vi "Ohaus (com6).vi"(4 "State":i16, 5 "Time":dbl format="%.2f", 6 "Sensor Values":dbl[](array[numeric]), 7 "Set Points":dbl[](array[numeric])) -> (0 "required data":T1, 3 "output value":dbl)   [LabVIEW 2015]
uses:
  <vilib>/Instr/_visa.llb/VISA Configure Serial Port (Instr).vi
panel:
  out "VISA resource name out":refnum<visa-resource-name>
  # "Enter the correct information for this control code in the required data structure below. Then make the current value default by right clicking on the border of the data structure. Select \"data operations\" and then select \"make current value default\". These values will be displayed by process controller."
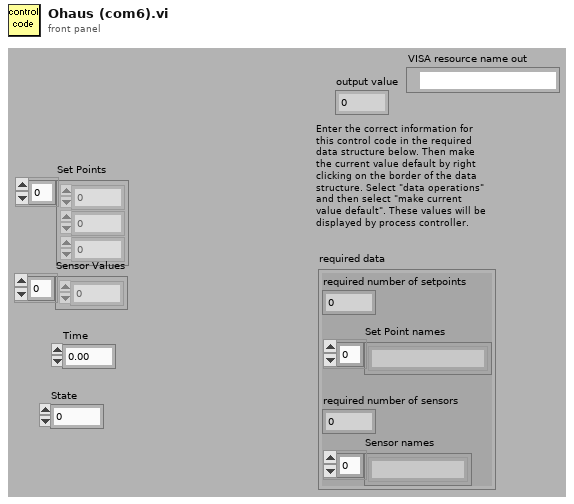
[diagram p1: front panel]
types:
  T1 = cluster{"Set Point names":string[], "required number of setpoints":u8, "required number of sensors":u8, "Sensor names":string[]}
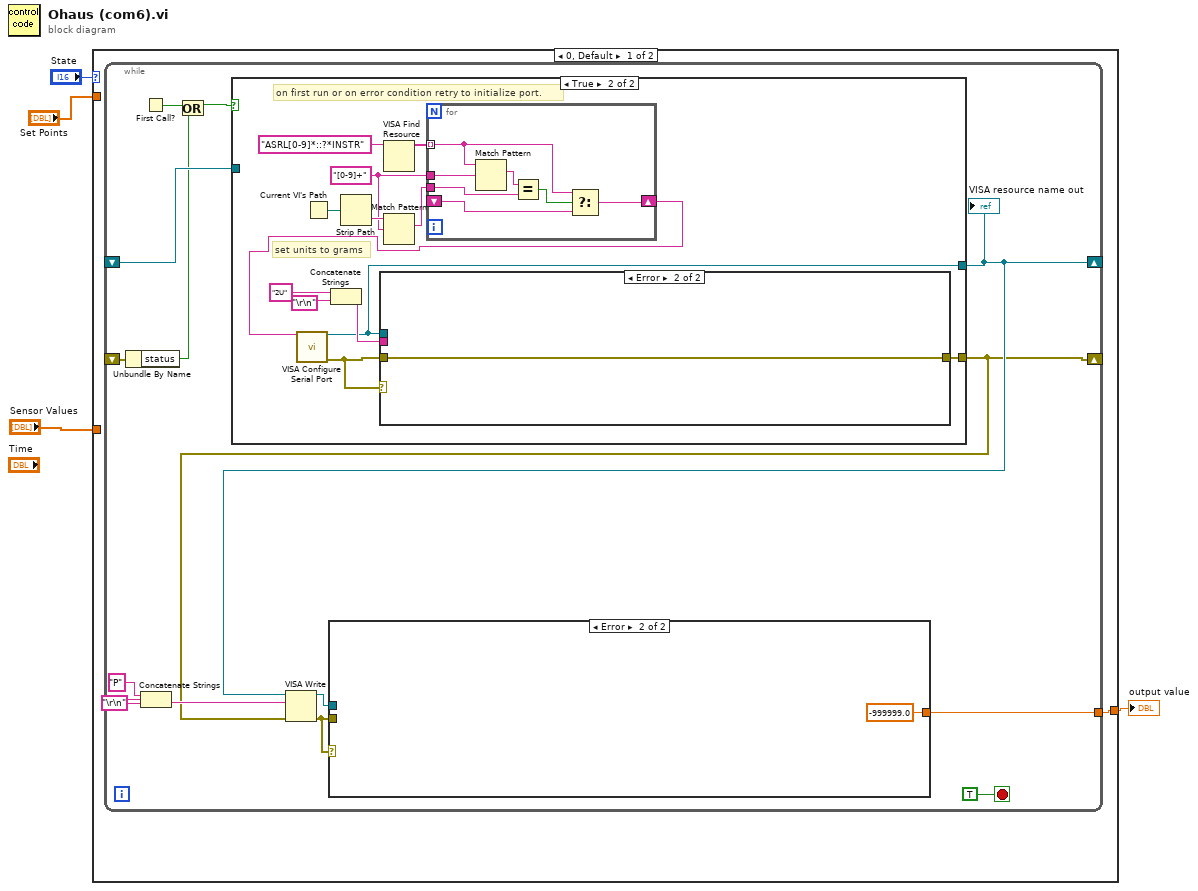
[diagram p0: block diagram]
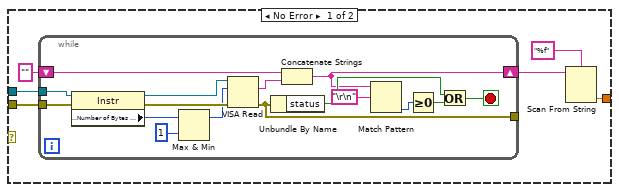
[diagram p2: hidden frame]
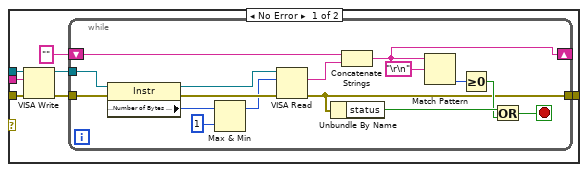
[diagram p4: hidden frame]
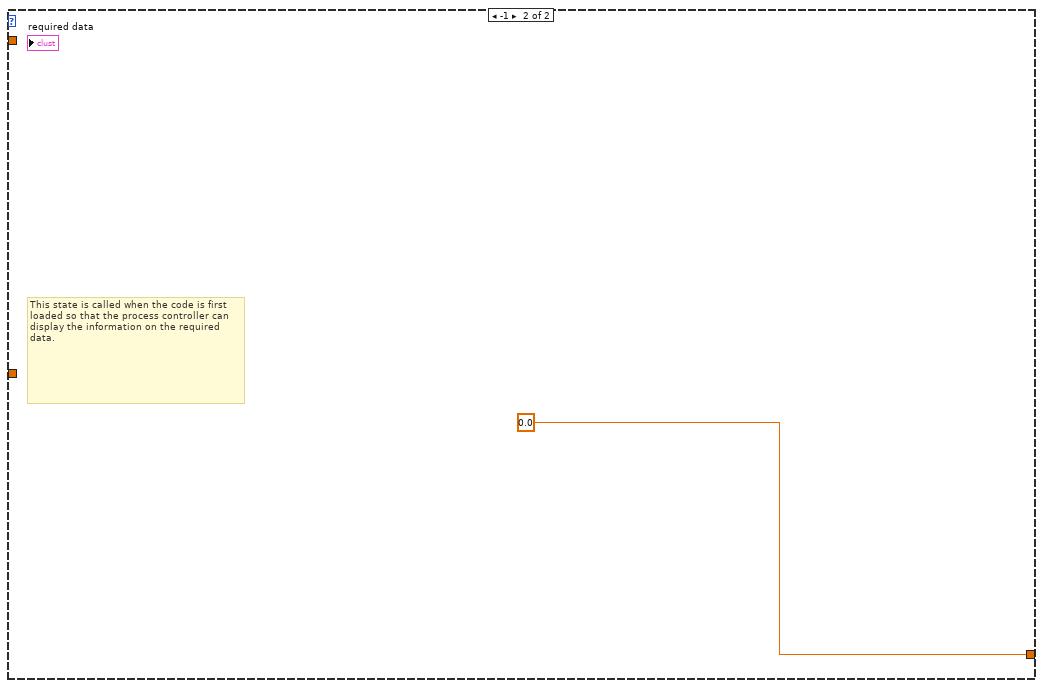
[diagram p5: hidden frame]
diagram:
  n1 = case shown="0, Default" "State" {
    tunnel: [w5 0.0 ("fraction on")] -> w3
    tunnel: "Set Points" -> [_ _]
    tunnel: "Sensor Values" -> [_ _]
    frame 0, Default {
      n2 = while {
        tunnel: [w19] -> w5
        shift-right: [w12] -> _
        shift-left: _ -> [w13]
        shift-right: [w10] -> _
        shift-left: _ -> [w9]
        stop <- TRUE stop-if-true
        n3 = Unbundle By Name(w9) -> ("status"=w7:bool)
        n4 = First Call?() -> (First Call?: T/F=w17:bool)
        n5 = Concatenate Strings("P", "\r\n") -> (w14:string)
        n6 = Or(x=w17, y=w7) -> (x .or. y?=w8:bool)
        n7 = case shown="True" w8 {
          tunnel: [_ w53] -> w10
          tunnel: [w43 w45] -> w12
          tunnel: w13 -> [w43 _]
          frame False {
          }
          frame True {
            w47 = "[0-9]+" ("regular expression")
            # "on first run or on error condition retry to initialize port."
            # "set units to grams"
            n8 = Current VI's Path() -> (path=w52:path)
            n9 = Concatenate Strings("2U", "\r\n") -> (w54:string)
            n10 = Strip Path(path=w52) -> (name=w51:string)  [unwired: 1 out]
            n11 = VISA Find Resource(11:"ASRL[0-9]*::?*INSTR" ("expression (\"?*\")")) -> (3:w49:string[])  [unwired: 2 in, 2 out]
            n12 = Match Pattern(string=w51, regular expression=w47) -> (match substring=w48:string)  [unwired: 1 in, 3 out]
            n13 = for {
              tunnel: w49 -> [w82] mode=indexing
              tunnel: w48 -> [w86]
              shift-right: [w83] -> w46
              shift-left: _ -> [w84]
              tunnel: w47 -> [w81]
              n14 = Match Pattern(string=w82, regular expression=w81) -> (match substring=w87:string)  [unwired: 1 in, 3 out]
              n15 = Equal?(x=w87, y=w86) -> (x = y?=w85:bool)
              n16 = Select(t=w82, s=w85, f=w84) -> (s? t:f=w83:string)
            }
            n17 = call-poly "VISA Configure Serial Port"("VISA resource name"=w46) -> ("VISA resource name out"=w45:refnum<visa-resource-name>, "error out"=w44:errorcluster)  [unwired: 13 in]
            n18 = case shown="Error" w44 {
              tunnel: w54 -> [w61 _]
              tunnel: w44 -> [w60 w80]
              tunnel: [w58 w80] -> w53
              tunnel: w45 -> [w57 _]
              frame No Error {
                n19 = VISA Write(VISA resource name=w57, write buffer=w61, error in (no error)=w60) -> (VISA resource name out=w59:refnum<visa-resource-name>, error out=w63:errorcluster)  [unwired: 1 out]
                n20 = while {
                  tunnel: w59 -> [w78]
                  tunnel: w63 -> [w76]
                  shift-right: [w64] -> _
                  shift-left: "" ("write buffer") -> [w79]
                  tunnel: [w65] -> w58
                  stop <- w74 stop-if-true
                  n21 = property class="Instr"(reference=w78, error in=w76) -> (reference out=w77:refnum<visa-resource-name>, error out=w75:errorcluster, "Serial Settings:Number of Bytes at Serial Port"=w67:u32)
                  n22 = Max & Min(x=w67, y=u32 1) -> (max(x,y)=w68:u32)  [unwired: 1 out]
                  n23 = VISA Read(VISA resource name=w77, byte count=w68, error in (no error)=w75) -> (read buffer=w72:string, error out=w65:errorcluster)  [unwired: 2 out]
                  n24 = Unbundle By Name(w65) -> ("status"=w73:bool)
                  n25 = Concatenate Strings(w79, w72) -> (w64:string)
                  n26 = Match Pattern(string=w64, regular expression="\r\n") -> (offset past match=w70:i32)  [unwired: 1 in, 3 out]
                  n27 = Greater Or Equal To 0?(x=w70) -> (x >= 0?=w69:bool)
                  n28 = Or(x=w73, y=w69) -> (x .or. y?=w74:bool)
                }
              }
              frame Error {
              }
            }
          }
        }
        "VISA resource name out" <- w12
        n29 = VISA Write(VISA resource name=w12, write buffer=w14, error in (no error)=w10) -> (VISA resource name out=w18:refnum<visa-resource-name>, error out=w6:errorcluster)  [unwired: 1 out]
        n30 = case shown="Error" w6 {
          tunnel: [w25 -999999.0] -> w19
          tunnel: w18 -> [w24 _]
          tunnel: w6 -> [w23 _]
          frame No Error {
            n31 = while {
              tunnel: w24 -> [w40]
              tunnel: w23 -> [w38]
              shift-right: [w26] -> w20
              shift-left: "" ("write buffer") -> [w41]
              tunnel: [w27] -> _
              stop <- w36 stop-if-true
              n32 = property class="Instr"(reference=w40, error in=w38) -> (reference out=w39:refnum<visa-resource-name>, error out=w37:errorcluster, "Serial Settings:Number of Bytes at Serial Port"=w29:u32)
              n33 = Max & Min(x=w29, y=u32 1) -> (max(x,y)=w30:u32)  [unwired: 1 out]
              n34 = VISA Read(VISA resource name=w39, byte count=w30, error in (no error)=w37) -> (read buffer=w34:string, error out=w27:errorcluster)  [unwired: 2 out]
              n35 = Unbundle By Name(w27) -> ("status"=w35:bool)
              n36 = Concatenate Strings(w41, w34) -> (w26:string)
              n37 = Match Pattern(string=w26, regular expression="\r\n") -> (offset past match=w32:i32)  [unwired: 1 in, 3 out]
              n38 = Greater Or Equal To 0?(x=w32) -> (x >= 0?=w31:bool)
              n39 = Or(x=w35, y=w31) -> (x .or. y?=w36:bool)
            }
            n40 = Scan From String(format string="%f", input string=w20) -> (output 1=w25:dbl)  [unwired: 3 in, 3 out]
          }
          frame Error {
          }
        }
      }
    }
    frame -1 {
      # "This state is called when the code is first loaded so that the process controller can display the information on the required data."
    }
  }
  "output value" <- w3
